vi "Option Parser.vi"(0 "Universal Power Meter in":refnum<class "Universal Power Meter.lvclass">, 1 "ID":string, 2 "THD?":bool, 3 "Number of Cards":dbl, 4 "ID cluster.Model":string, 5 "error in (no error)":errorcluster, 7 "Option":string) -> (14 "Universal Power Meter out":refnum<class "Universal Power Meter.lvclass">, 19 "error out":errorcluster)   [LabVIEW 2014, in "Universal Power Meter.lvlib" / "Universal Power Meter.lvclass"]
uses:
  Universal Power Meter.lvclass
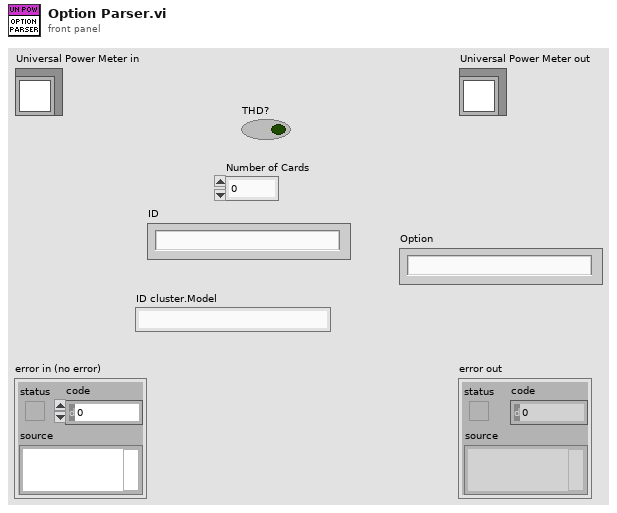
[diagram p1: front panel]
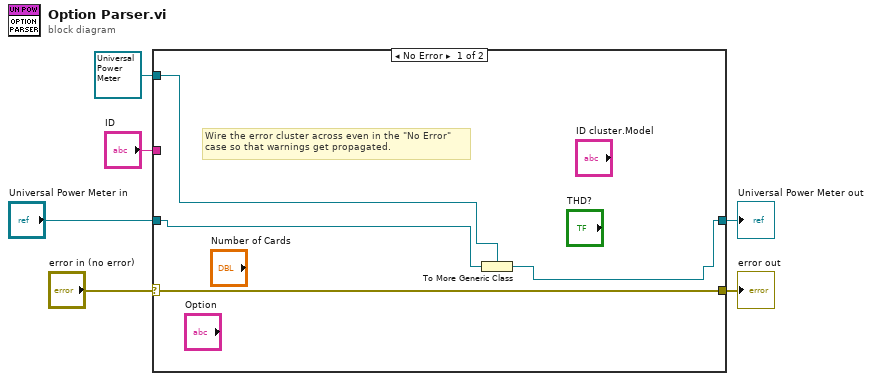
[diagram p0: block diagram]
diagram:
  n1 = case shown="No Error" "error in (no error)" {
    selector: "error in (no error)" -> [w7 w12]
    tunnel: [w7 w12] -> w5
    tunnel: [w8 w11] -> w3
    tunnel: "Universal Power Meter in" -> [w10 w11]
    tunnel: refnum<class "Universal Power Meter.lvclass"> refnum ("Universal Power Meter.lvlib:Universal Power Meter.lvclass") -> [w9 _]
    tunnel: "ID" -> [_ _]
    frame No Error {
      # "Wire the error cluster across even in the \"No Error\"\ncase so that warnings get propagated."
      n2 = To More Generic Class(target class=w9, reference=w10) -> (generic class reference=w8:refnum<class "Universal Power Meter.lvclass">)
    }
    frame Error {
    }
  }
  "error out" <- w5
  "Universal Power Meter out" <- w3
